vi "tb_FFT Output_Ping Pong BRAM.vi"() -> ()   [LabVIEW 2011]
panel:
  out "Address 2":dbl[](array[numeric])
  out "Address 1":dbl[](array[numeric])
  out "Data 2":dbl[](array[numeric])
  in  "Ticks":i32=4
  out "Data1":dbl[](array[numeric])
  in  "Iterations":i32=100
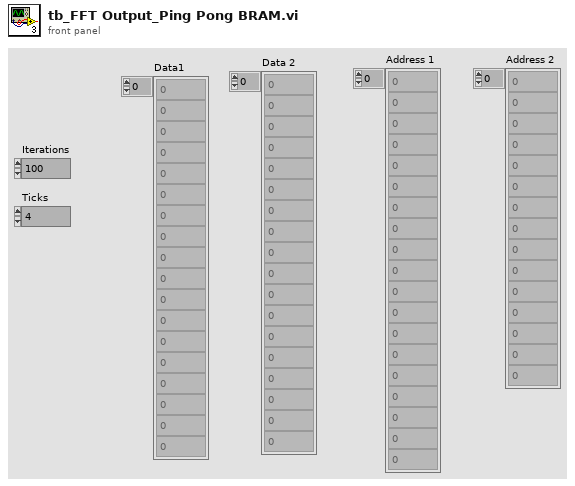
[diagram p1: front panel]
types:
  T1 = cluster{"Data 1":u64, "Data Valid 1":bool, "Address1":u16}
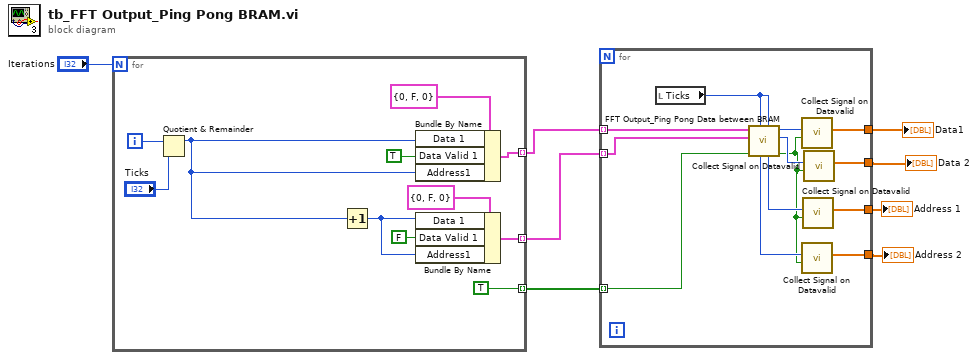
[diagram p0: block diagram]
diagram:
  n1 = for {
    N: "Iterations" -> [_]
    tunnel: [w18] -> w7 mode=indexing
    tunnel: [w15] -> w6 mode=indexing
    tunnel: [TRUE] -> w5 mode=indexing
    i -> [w12]
    n2 = Quotient & Remainder(x=w12, y="Ticks") -> (x-y*floor(x/y)=w9:i32)  [unwired: 1 out]
    n3 = Increment(x=w9) -> (x+1=w10:i32)
    n4 = Bundle By Name(cluster=T1 {"Data 1"=0, "Data Valid 1"=FALSE, "Address1"=0} ("Bank0 Data"), "Data 1"=w9, "Data Valid 1"=TRUE, "Address1"=w9) -> (w18:T1)
    n5 = Bundle By Name(cluster=T1 {"Data 1"=0, "Data Valid 1"=FALSE, "Address1"=0} ("Bank0 Data"), "Data 1"=w10, "Data Valid 1"=FALSE, "Address1"=w10) -> (w15:T1)
  }
  n6 = for {
    tunnel: w7 -> [w32] mode=indexing
    tunnel: w6 -> [w31] mode=indexing
    tunnel: w5 -> [w30] mode=indexing
    tunnel: [w27] -> w4
    tunnel: [w26] -> w3
    tunnel: [w22] -> w2
    tunnel: [w21] -> w1
    n7 = local read "Ticks"() -> (w20:i32)
    n8 = call <userlib>:"FFT Output_Ping Pong Data between BRAM.vi"("Read Count"=w20, "Write Count"=w20, "Input Valid"=w30, "Bank1 Data"=w31, "Bank0 Data"=w32) -> ("Read Valid"=w23:bool, "Address1. Element Out"=w28:u16, "Address0. Element Out"=w29:u16, "Read Address 1"=w25:u16, "Read Address 0"=w24:u16)  [unwired: 2 in]
    n9 = call <userlib>:"Collect Signal on Datavalid.vi"("Data Valid"=w23, "Input"=w29) -> ("Output"=w27:dbl[])  [unwired: 9 in]
    n10 = call <userlib>:"Collect Signal on Datavalid.vi"("Data Valid"=w23, "Input"=w24) -> ("Output"=w21:dbl[])  [unwired: 9 in]
    n11 = call <userlib>:"Collect Signal on Datavalid.vi"("Data Valid"=w23, "Input"=w25) -> ("Output"=w22:dbl[])  [unwired: 9 in]
    n12 = call <userlib>:"Collect Signal on Datavalid.vi"("Data Valid"=w23, "Input"=w28) -> ("Output"=w26:dbl[])  [unwired: 9 in]
  }
  "Data1" <- w4
  "Data 2" <- w3
  "Address 1" <- w2
  "Address 2" <- w1
